vi "JVCurveParameters_Aging_Martina.vi"(1 "Cell to be measured In":T2) -> (0 "Measurements Out":T1)   [LabVIEW 2011]
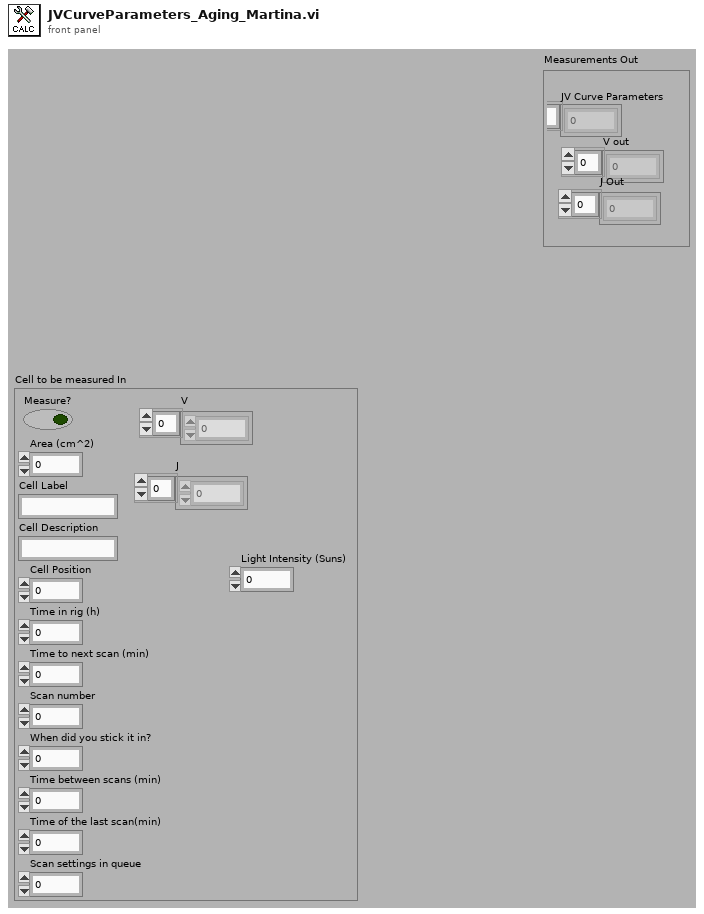
[diagram p1: front panel]
types:
  T1 = cluster{"JV Curve Parameters":dbl[], "V out":dbl[], "J Out":dbl[]}
  T2 = cluster{"Measure?":bool, "Area (cm^2)":dbl, "Cell Label":string, "Cell Description":string, "Cell Position":i32, "Time in rig (h)":dbl, "Time to next scan (min)":dbl, "Scan number":dbl, "When did you stick it in?":dbl, "Time between scans (min)":dbl, "Time of the last scan(min)":dbl, "Scan settings in queue":u16, "V":dbl[], "J":dbl[], "Light Intensity (Suns)":dbl}
  T3 = cluster{"JV Curve Parameters 2":dbl[], "V out":dbl[], "J Out":dbl[]}
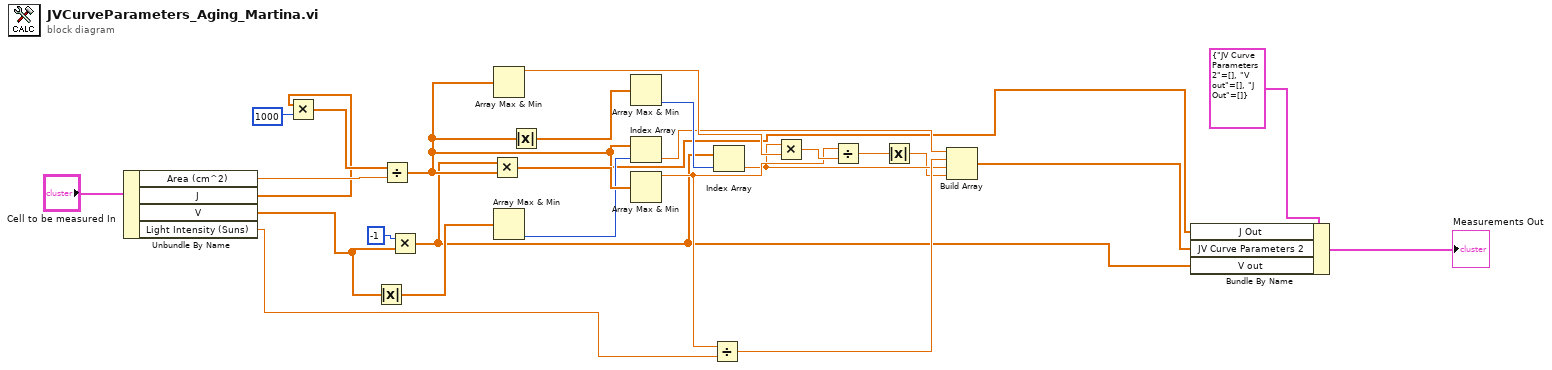
[diagram p0: block diagram]
diagram:
  n1 = Unbundle By Name("Cell to be measured In") -> ("Area (cm^2)"=w4:dbl, "J"=w3:dbl[], "V"=w2:dbl[], "Light Intensity (Suns)"=w1:dbl)
  n2 = Multiply(x=w3, y=1000) -> (x*y=w18:dbl[])
  n3 = Absolute Value(x=w2) -> (abs(x)=w13:dbl[])
  n4 = Divide(x=w18, y=w4) -> (x/y=w7:dbl[])
  n5 = Multiply(x=-1, y=w2) -> (x*y=w5:dbl[])
  n6 = Multiply(x=w5, y=w7) -> (x*y=w21:dbl[])
  n7 = Array Max & Min(array=w7) -> (max value=w17:dbl)  [unwired: 3 out]
  n8 = Array Max & Min(array=w13) -> (min index (indices)=w12:i32)  [unwired: 3 out]
  n9 = Absolute Value(x=w7) -> (abs(x)=w24:dbl[])
  n10 = Array Max & Min(array=w24) -> (min index (indices)=w23:i32)  [unwired: 3 out]
  n11 = Index Array(array=w7, index=w12) -> (element=w11:dbl)
  n12 = Array Max & Min(array=w21) -> (max value=w20:dbl)  [unwired: 3 out]
  n13 = Divide(x=w20, y=w1) -> (x/y=w16:dbl)
  n14 = Index Array(array=w5, index=w23) -> (element=w15:dbl)
  n15 = Multiply(x=w15, y=w17) -> (x*y=w22:dbl)
  n16 = Divide(x=w20, y=w22) -> (x/y=w25:dbl)
  n17 = Absolute Value(x=w25) -> (abs(x)=w14:dbl)
  n18 = Build Array(w11, w16, w15, w14) -> (w6:dbl[])
  n19 = Bundle By Name(cluster=T3 {"JV Curve Parameters 2"=[], "V out"=[], "J Out"=[]} ("Cluster"), "J Out"=w7, "JV Curve Parameters 2"=w6, "V out"=w5) -> (→"Measurements Out":T3)
